vi "Get JSON File Path.vi"(8 "error in (no error)":errorcluster, 10 "Slot #":i32=1, 11 "Slot 1 Module Type":T1) -> (0 "error out":errorcluster, 3 "appended path":path)   [LabVIEW 2017]
uses:
  Module Type.ctl
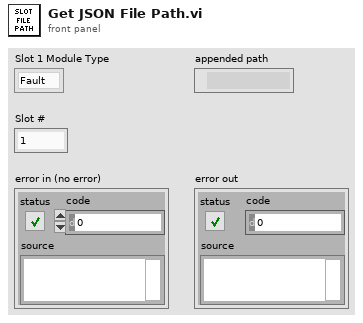
[diagram p1: front panel]
types:
  T1 = typedef "Module Type.ctl" = enum16{"Fault", "Instrument"}
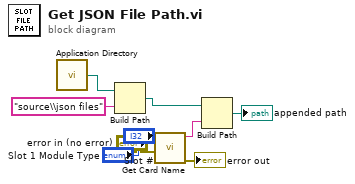
[diagram p0: block diagram]
diagram:
  n1 = call <vilib>:"Application Directory.vi"() -> ("Application Directory"=w3:path)
  n2 = Build Path(base path=w3, name or relative path="source\\json files") -> (appended path=w5:path)
  n3 = call "Get Card Name.vi"("error in (no error)"="error in (no error)", "Slot #"="Slot #", "Slot 1 Module Type"="Slot 1 Module Type") -> ("error out"=→"error out":errorcluster, "resulting string"=w6:string)  [unwired: 7 in]
  n4 = Build Path(base path=w5, name or relative path=w6) -> (appended path=→"appended path":path)
